vi "instrumentProperties_channel_PD tempVariable.vi"(8 "error in (no error)":errorcluster, 11 "OSAchannel in":refnum<class "OSAchannel.lvclass">) -> (0 "error out":errorcluster, 2 "tempVar_available":bool, 3 "OSAchannel out":refnum<class "OSAchannel.lvclass">)   [LabVIEW 2010, in "OSAchannel.lvclass"]
uses:
  OSAchannel.lvclass
  OSAchannel.lvclass/OSAchannel.ctl
  _dll/LVLib/FTSLib.lvlib
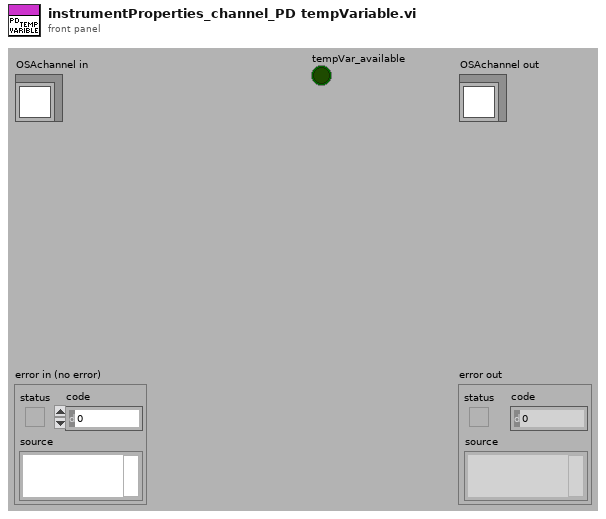
[diagram p1: front panel]
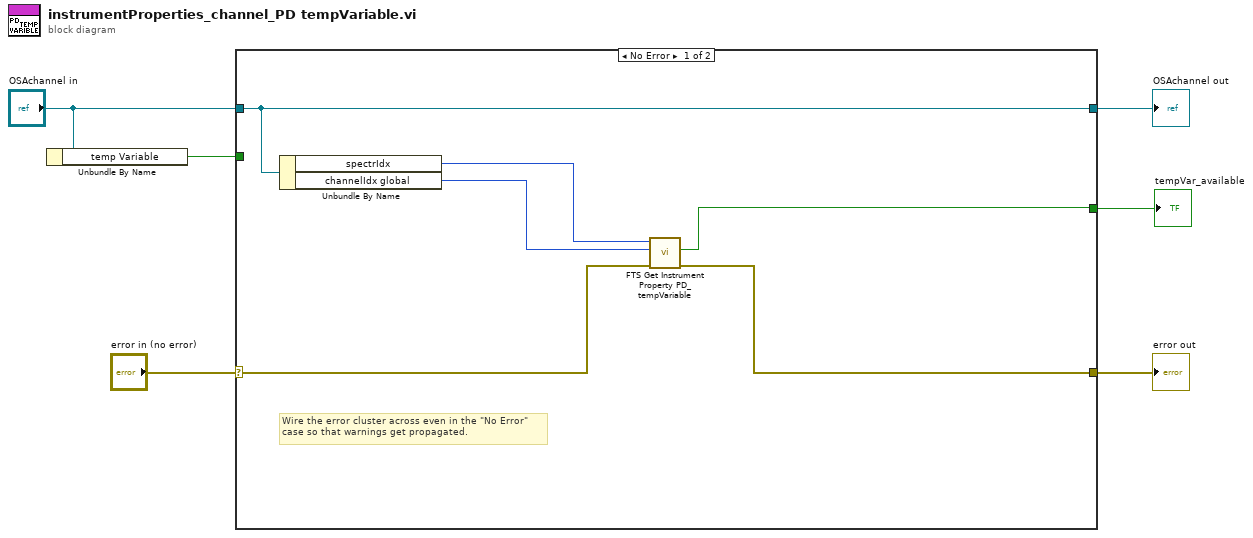
[diagram p0: block diagram]
diagram:
  n1 = Unbundle By Name("OSAchannel in") -> ("temp Variable"=w1:bool)
  n2 = case shown="No Error" "error in (no error)" {
    selector: "error in (no error)" -> [w9 w15]
    tunnel: [w8 w15] -> w5
    tunnel: [w12 w14] -> w4
    tunnel: "OSAchannel in" -> [w12 w14]
    tunnel: [w7 w13] -> w3
    tunnel: w1 -> [_ w13]
    frame No Error {
      # "Wire the error cluster across even in the \"No Error\"\ncase so that warnings get propagated."
      n3 = Unbundle By Name(w12) -> ("spectrIdx"=w11:u16, "channelIdx global"=w10:u16)
      n4 = call "FTS Get Instrument Property PD_tempVariable.vi"("error in (no error)"=w9, "channel"=w10, "spectrIdx"=w11) -> ("error out"=w8:errorcluster, "tempVar_available"=w7:bool)  [unwired: 7 in]
    }
    frame Error {
    }
  }
  "error out" <- w5
  "OSAchannel out" <- w4
  "tempVar_available" <- w3
